vi "MT Apply Pulse Shaping Filter (FSK).vi"(0 "symbols":dbl[](array[numeric]) min=0.0 max=127.0 format="%.2f", 5 "pulse shaping filter coefficients":dbl[](array[numeric]) format="%.2f", 7 "samples per symbol (16)":i32=16, 9 "symbol rate (Hz)":dbl=1.0, 11 "error in (no error)":errorcluster, 12 "symbol phase continuity":enum16{"continuous", "discontinuous"}(ring), 13 "reset? (T)":bool=TRUE) -> (4 "output phase waveform":cluster{"t0":dbl, "dt":dbl, "Y":cdb[]}={"t0"=0.0, "dt"=1.0, "Y"=[]} {"Y" format="%.3f"; "dt" format="%^.2e"; "t0" format="%.4f"}, 15 "error out":errorcluster)   [LabVIEW 2020, in "niDMT.lvlib"]
doc: "This polymorphic instance applies a pulse-shaping filter to an input stream comprised of FSK-modulated symbols. The VI performs filtering using the specified <B>pulse shaping filter coefficients</B> followed by accumulation on the phase of the information symbols to generate the oversampled FSK-modulated complex baseband waveform. This process is the digital equivalent of continuous-time analog frequency modulation.\n\n<B>NOTE:</B> If you set the"
uses:
  <vilib>/addons/Modulation/niDMT.lvlib
  <vilib>/addons/Modulation/niAMT.lvlib
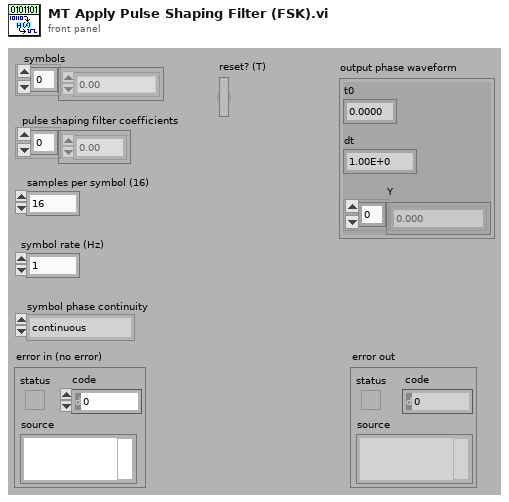
[diagram p1: front panel]
types:
  T1 = typedef "niAMT.lvlib/Complex Data Waveform.ctl" = cluster{"t0":dbl, "dt":dbl, "Y":cdb[]}
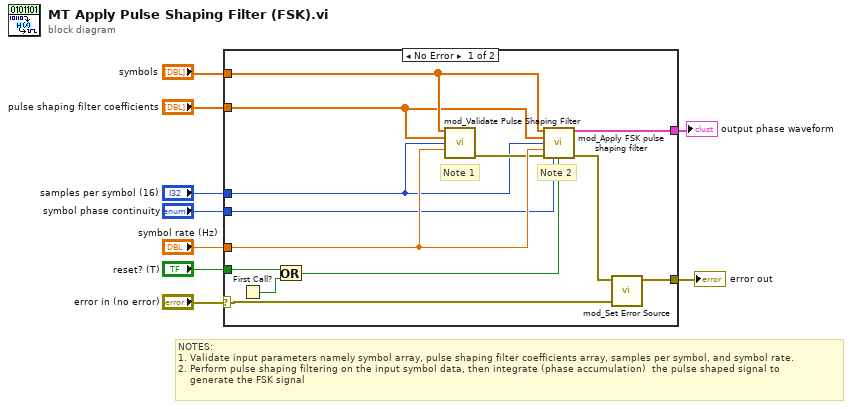
[diagram p0: block diagram]
diagram:
  # "NOTES:\n1. Validate input parameters namely symbol array, pulse shaping filter coefficients array, samples per symbol, and symbol rate.\n2. Perform pulse shaping filtering on the input symbol data, then integrate (phase accumulation)  the pulse shaped signal to \n    generate the FSK signal"
  n1 = case shown="No Error" "error in (no error)" {
    selector: "error in (no error)" -> [w13 w23]
    tunnel: "symbols" -> [w18 _]
    tunnel: "pulse shaping filter coefficients" -> [w17 _]
    tunnel: "symbol rate (Hz)" -> [w16 _]
    tunnel: "reset? (T)" -> [w21 _]
    tunnel: [w19 _] -> w4
    tunnel: [w12 w23] -> w3
    tunnel: "samples per symbol (16)" -> [w11 _]
    tunnel: "symbol phase continuity" -> [w10 _]
    frame No Error {
      # "Note 2"
      # "Note 1"
      n2 = First Call?() -> (First Call?: T/F=w20:bool)
      n3 = Or(x=w21, y=w20) -> (x .or. y?=w22:bool)
      n4 = call <vilib>:"mod_Validate Pulse Shaping Filter.vi"("symbols"=w18, "pulse shaping filter coefficients"=w17, "samples per symbol (16)"=w11, "symbol Rate, Hz"=w16) -> ("error out"=w15:errorcluster)  [unwired: 11 out]
      n5 = call <vilib>:"mod_Apply FSK pulse shaping filter.vi"("symbols"=w18, "pulse shaping filter coefficients"=w17, "samples per symbol (16)"=w11, "symbol rate"=w16, "error in (no error)"=w15, "symbol phase continuity"=w10, "reset? (T)"=w22) -> ("output complex waveform"=w19:T1, "error out"=w14:errorcluster)  [unwired: 7 out]
      n6 = call <vilib>:"mod_Set Error Source.vi"("initial error in (no error)"=w13, "final error in (no error)"=w14) -> ("error out"=w12:errorcluster)  [unwired: 3 out]
    }
    frame Error {
    }
  }
  "output phase waveform" <- w4
  "error out" <- w3
